vi "OpenSystemDefinitionFile.vi"(8 "error in (no error)":errorcluster, 11 "VeriStand Test Case in":refnum<class "VeriStandTestCase.lvclass">) -> (0 "error out":errorcluster, 3 "VeriStand Test Case out":refnum<class "VeriStandTestCase.lvclass">)   [LabVIEW 2027, in "VeriStandTestCase.lvclass"]
uses:
  VeriStandTestCase.lvclass
  VeriStandTestCase.lvclass/VeriStandTestCase.ctl
  <vilib>/NI VeriStand/Execution/Workspace/NI_VS Workspace ExecutionAPI.lvlib
  VeriStandTestUtilities/VeriStandTestUtilities.lvlib
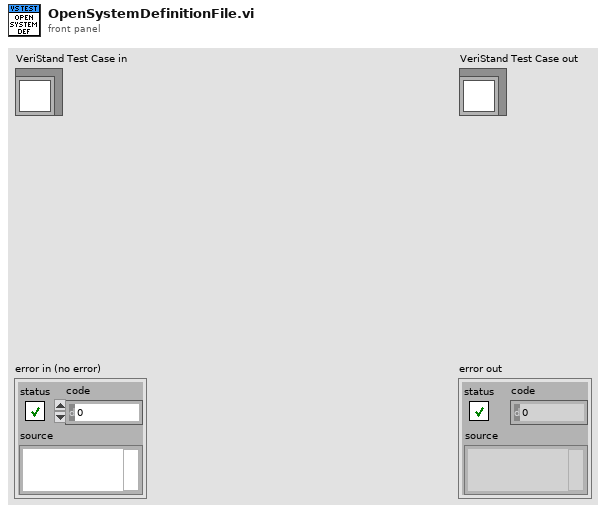
[diagram p1: front panel]
types:
  T1 = typedef "NI_VS Workspace ExecutionAPI.lvlib/WorkspaceAPI.ctl" = refnum<k39>
  T2 = typedef "VeriStandTestUtilities.lvlib/SystemDefinitionInformation.ctl" = cluster{"Path":path, "Target Information List":T3[]}
  T3 = typedef "VeriStandTestUtilities.lvlib/TargetInformation.ctl" = cluster{"Name":string, "IP Address":string, "Operating System":string, "Target Rate":dbl, "Chassis List":T4[], "Custom Device List":string[]}
  T4 = typedef "VeriStandTestUtilities.lvlib/ChassisInformation.ctl" = cluster{"Name":string, "Devices":string[]}
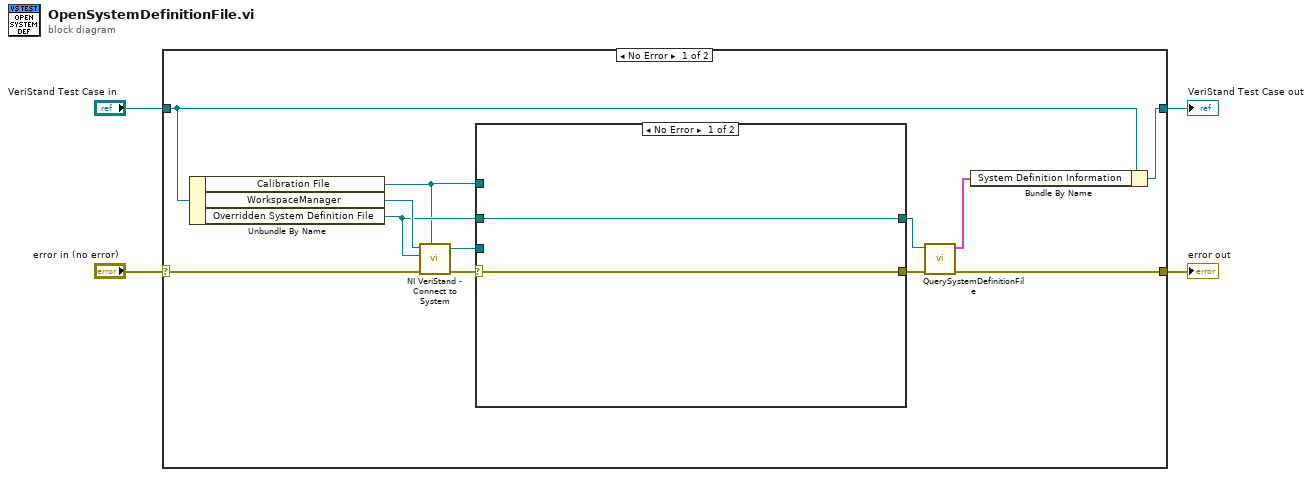
[diagram p0: block diagram]
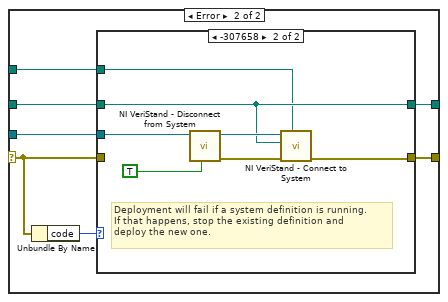
[diagram p2: hidden frame]
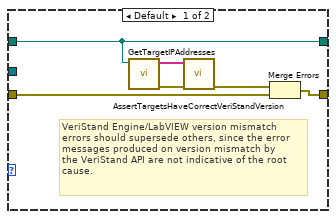
[diagram p3: hidden frame]
diagram:
  n1 = case shown="No Error" "error in (no error)" {
    selector: "error in (no error)" -> [w14 w40]
    tunnel: [w9 w40] -> w4
    tunnel: [w10 w39] -> w2
    tunnel: "VeriStand Test Case in" -> [w11 w39]
    frame No Error {
      n2 = Unbundle By Name(w11) -> ("Calibration File"=w5:path, "WorkspaceManager"=w15:T1, "Overridden System Definition File"=w6:path)
      n3 = call <vilib>:"NI VeriStand - Connect to System.vi"("Calibration File"=w5, "error in (no error)"=w14, "System Definition File (.nivssdf)"=w6, "WorkspaceManager in"=w15) -> ("error out"=w13:errorcluster, "WorkspaceManager out"=w12:T1)  [unwired: 6 in]
      n4 = case shown="No Error" w13 {
        selector: w13 -> [w18 w22]
        tunnel: [w18 w25] -> w16
        tunnel: w6 -> [w17 w24]
        tunnel: w12 -> [_ w23]
        tunnel: [w17 w20] -> w8
        tunnel: w5 -> [_ w19]
        frame No Error {
        }
        frame Error {
          n5 = Unbundle By Name(w22) -> ("code"=w21:i32)
          n6 = case shown="-307658" w21 {
            tunnel: w22 -> [w29 _]
            tunnel: [w31 w38] -> w25
            tunnel: w23 -> [_ w36]
            tunnel: w24 -> [w26 w33]
            tunnel: [w26 w33] -> w20
            tunnel: w19 -> [_ w32]
            frame Default {
              # "VeriStand Engine/LabVIEW version mismatch\nerrors should supersede others, since the error\nmessages produced on version mismatch by\nthe VeriStand API are not indicative of the root\ncause."
              n7 = call "GetTargetIPAddresses.vi"("absolute system definition file"=w26) -> ("error out"=w27:errorcluster, "ip addresses"=w28:string[])  [unwired: 9 in]
              n8 = call "AssertTargetsHaveCorrectVeriStandVersion.vi"("error in (no error)"=w27, "targets"=w28) -> ("error out"=w30:errorcluster)  [unwired: 9 in]
              n9 = Merge Errors(w30, w29) -> (w31:errorcluster)
            }
            frame -307658 {
              # "Deployment will fail if a system definition is running.\nIf that happens, stop the existing definition and\ndeploy the new one."
              n10 = call <vilib>:"NI VeriStand - Disconnect from System.vi"("Undeploy System Definition (F)"=TRUE, "WorkspaceManager in"=w36) -> ("error out"=w37:errorcluster, "WorkspaceManager out"=w35:T1)  [unwired: 8 in]
              n11 = call <vilib>:"NI VeriStand - Connect to System.vi"("Calibration File"=w32, "error in (no error)"=w37, "System Definition File (.nivssdf)"=w33, "WorkspaceManager in"=w35) -> ("error out"=w38:errorcluster)  [unwired: 6 in, 1 out]
            }
          }
        }
      }
      n12 = call "QuerySystemDefinitionFile.vi"("error in (no error)"=w16, "System Definiton File in"=w8) -> ("error out"=w9:errorcluster, "System Definition Information out"=w7:T2)  [unwired: 8 in]
      n13 = Bundle By Name(cluster=w11, "System Definition Information"=w7) -> (w10:refnum<class "VeriStandTestCase.lvclass">)
    }
    frame Error {
    }
  }
  "error out" <- w4
  "VeriStand Test Case out" <- w2
